vi "Authenticated.vi"(7 "Address":string, 8 "Error In":errorcluster) -> (0 "Error Out":errorcluster)   [LabVIEW 2018, in "Tests.lvlib" / "Session.lvlib"]
uses:
  Session.lvlib
  <vilib>/addons/_JKI Toolkits/Caraya/classes/Test/Test.lvclass
  src/Toolkit/SSH/SSH.lvclass
  src/Toolkit/Session/Session.lvclass
  <vilib>/addons/_JKI Toolkits/Caraya/classes/Assert/Assert.lvclass
  Tests.lvlib
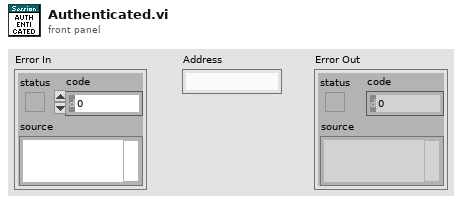
[diagram p1: front panel]
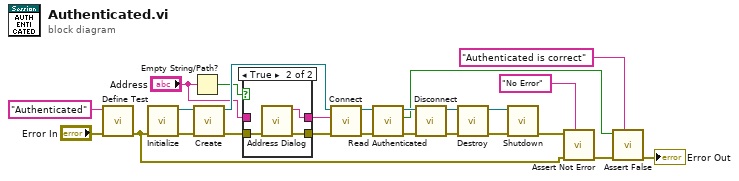
[diagram p0: block diagram]
diagram:
  n1 = call <vilib>:"Define Test.vi"("error in (no error)"="Error In", "Label (VI Title)"="Authenticated") -> ("error out"=w17:errorcluster)  [unwired: 9 in]
  n2 = call "Initialize.vi"("Error In"=w17) -> ("Error Out"=w23:errorcluster, "SSH"=w22:refnum<class "SSH.lvclass">)  [unwired: 9 in]
  n3 = Empty String/Path?(string/path="Address") -> (empty?=w5:bool)
  n4 = call "Create.vi"("Error In"=w23, "SSH"=w22) -> ("Error Out"=w4:errorcluster, "Sesssion"=w16:refnum<class "Session.lvclass">)  [unwired: 8 in]
  n5 = case shown="True" w5 {
    tunnel: w4 -> [w26 w30]
    tunnel: [w26 w29] -> w3
    tunnel: [w27 w28] -> w2
    tunnel: "Address" -> [w27 _]
    frame False {
    }
    frame True {
      n6 = call "Address Dialog.vi"("Error In"=w30) -> ("Error Out"=w29:errorcluster, "Address Out"=w28:string)  [unwired: 9 in]
    }
  }
  n7 = call "Connect.vi"("Error In"=w3, "Address"=w2, "Session In"=w16) -> ("Error Out"=w10:errorcluster, "Sesssion Out"=w11:refnum<class "Session.lvclass">)  [unwired: 7 in]
  n8 = call "Read Authenticated.vi"("Error In"=w10, "Session In"=w11) -> ("Error Out"=w9:errorcluster, "Authenticated"=w7:bool, "Sesssion Out"=w8:refnum<class "Session.lvclass">)  [unwired: 7 in]
  n9 = call "Disconnect.vi"("Error In"=w9, "Session In"=w8) -> ("Error Out"=w14:errorcluster, "Sesssion Out"=w15:refnum<class "Session.lvclass">)  [unwired: 8 in]
  n10 = call "Destroy.vi"("Error In"=w14, "Session"=w15) -> ("Error Out"=w20:errorcluster, "SSH"=w21:refnum<class "SSH.lvclass">)  [unwired: 8 in]
  n11 = call "Shutdown.vi"("Error In"=w20, "SSH"=w21) -> ("Error Out"=w19:errorcluster)  [unwired: 9 in]
  n12 = call <vilib>:"Assert Not Error.vi"("Label"="No Error", "error in (no error)"=w17, "Not Error?"=w19) -> ("error out"=w13:errorcluster)  [unwired: 8 in]
  n13 = call <vilib>:"Assert False.vi"("Label"="Authenticated is correct", "error in (no error)"=w13, "False?"=w7) -> ("error out"=→"Error Out":errorcluster)  [unwired: 8 in]
